vi "createPlatformDataV1.vi"() -> (3 "digital waveform":bool[](array[boolean]))   [LabVIEW 2017]
panel:
  in  "Select?":bool
  in  "Platform 61":bool
  in  "Platform 60":bool
  in  "Platform 59":bool
  in  "Platform 58":bool
  in  "Platform 57":bool
  in  "Platform 56":bool
  in  "Platform 55":bool
  in  "Platform 54":bool
  in  "Platform 53":bool
  in  "Platform 52":bool
  in  "Platform 51":bool
  in  "Platform 50":bool
  in  "Platform 49":bool
  in  "Platform 48":bool
  in  "Platform 47":bool
  in  "Platform 46":bool
  in  "Platform 45":bool
  in  "Platform 44":bool
  in  "Platform 43":bool
  in  "Platform 42":bool
  in  "Platform 41":bool
  in  "Platform 40":bool
  in  "Platform 39":bool
  in  "Platform 38":bool
  in  "Platform 37":bool
  in  "Platform 36":bool
  in  "Platform 35":bool
  in  "Platform 34":bool
  in  "Platform 33":bool
  in  "Platform 32":bool
  in  "Platform 31":bool
  in  "Platform 30":bool
  in  "Platform 29":bool
  in  "Platform 28":bool
  in  "Platform 27":bool
  in  "Platform 26":bool
  in  "Platform 25":bool
  in  "Platform 24":bool
  in  "Platform 23":bool
  in  "Platform 22":bool
  in  "Platform 21":bool
  in  "Platform 20":bool
  in  "Platform 19":bool
  in  "Platform 18":bool
  in  "Platform 17":bool
  in  "Platform 16":bool
  in  "Platform 15":bool
  in  "Platform 14":bool
  in  "Platform 13":bool
  in  "Platform 12":bool
  in  "Platform 11":bool
  in  "Platform 10":bool
  in  "Platform 9":bool
  in  "Platform 8":bool
  in  "Platform 7":bool
  in  "Platform 6":bool
  in  "Platform 5":bool
  in  "Platform 4":bool
  in  "Platform 3":bool
  in  "Platform 2":bool
  in  "Platform 1":bool
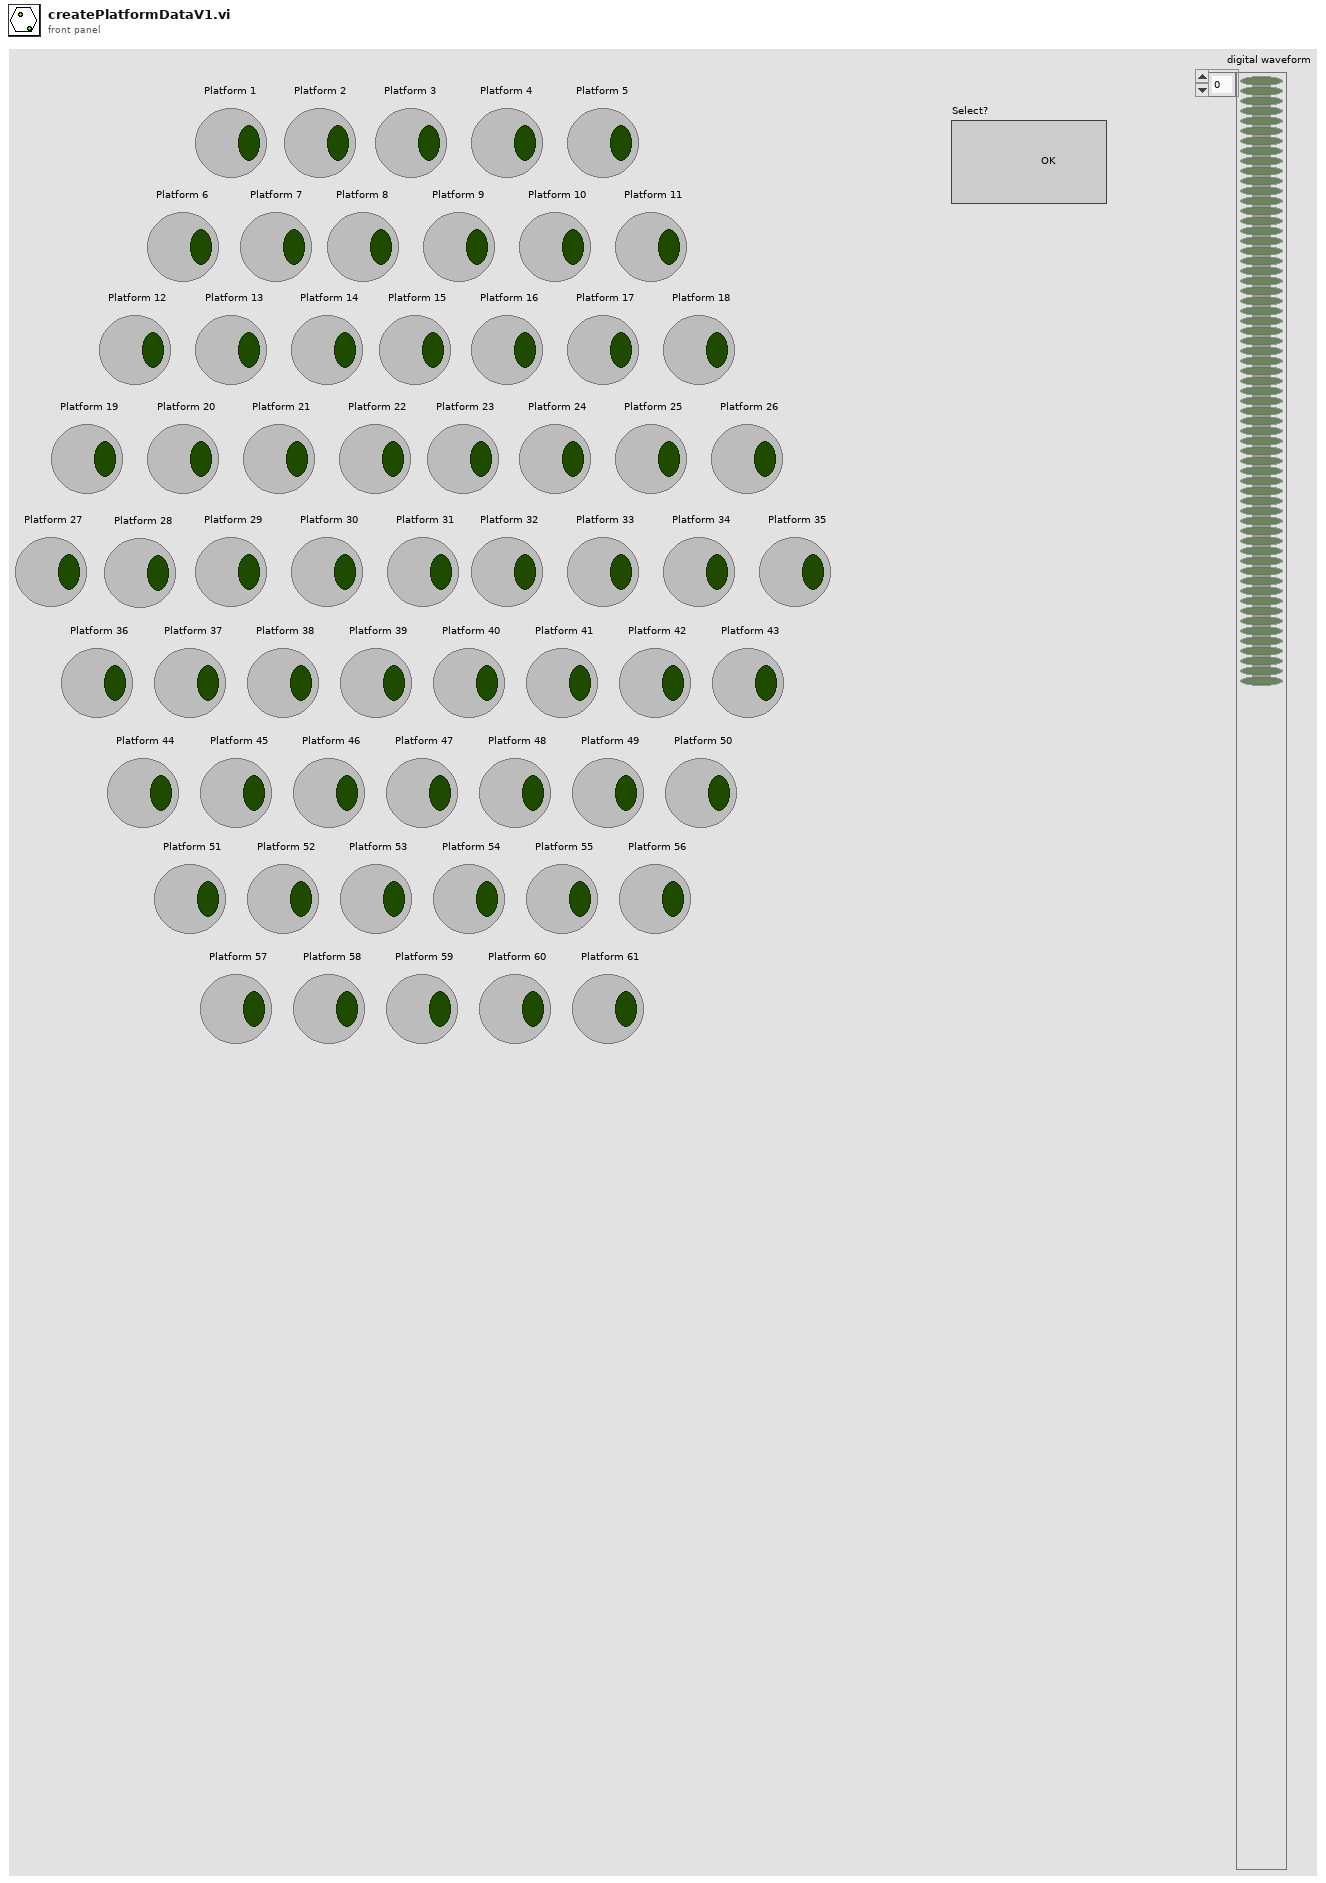
[diagram p1: front panel]
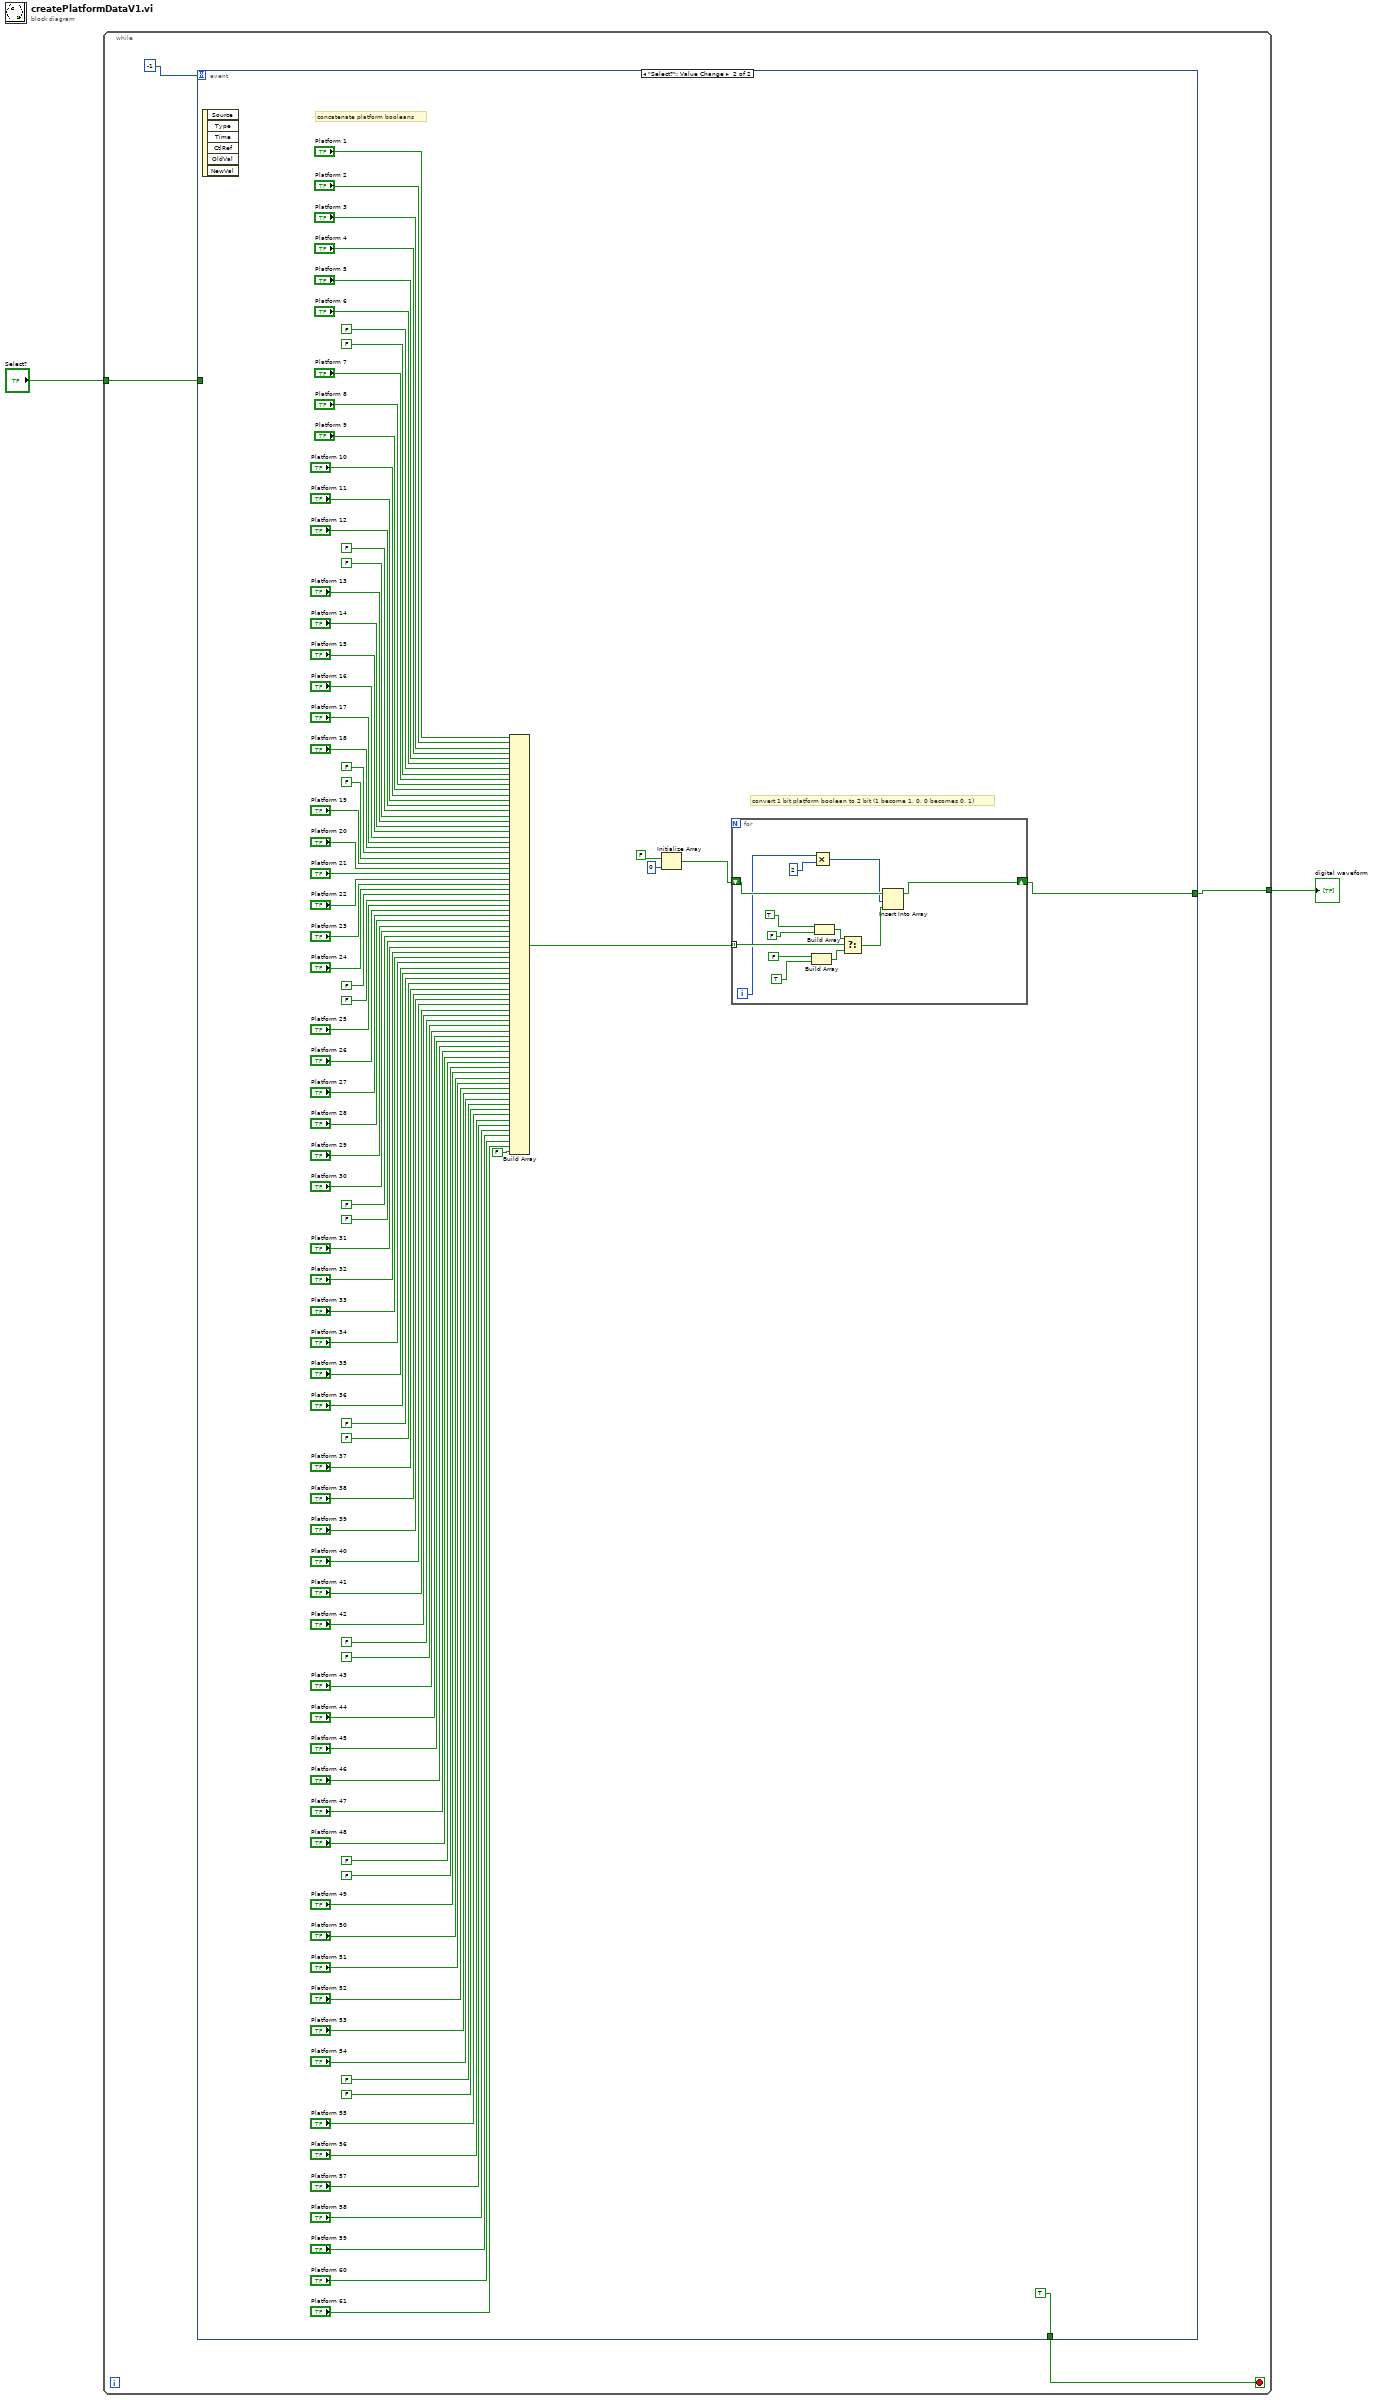
[diagram p0: block diagram]
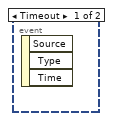
[diagram p2: hidden frame]
diagram:
  n1 = while {
    tunnel: "Select?" -> [w5]
    tunnel: [w3] -> w1
    stop <- w4 stop-if-true
    n2 = event shown="[1] \"Select?\": Value Change" {
      selector: _ -> [_ _]
      dyn-events: _ -> [_ _]
      timeout: -1 -> [_ _]
      tunnel: w5 -> [_ _]
      tunnel: [_ TRUE] -> w4
      tunnel: [_ w7] -> w3
      event Timeout {
        n3 = event-data() -> ()  [unwired: 1 in, 3 out]
      }
      event "Select?": Value Change {
        # "convert 1 bit platform boolean to 2 bit (1 become 1, 0, 0 becomes 0, 1)"
        # "concatenate platform booleans"
        n4 = event-data() -> ()  [unwired: 1 in, 6 out]
        n5 = Build Array("Platform 1", "Platform 2", "Platform 3", "Platform 4", "Platform 5", "Platform 6", FALSE, FALSE, "Platform 7", "Platform 8", "Platform 9", "Platform 10", "Platform 11", "Platform 12", FALSE, FALSE, "Platform 13", "Platform 14", "Platform 15", "Platform 16", "Platform 17", "Platform 18", FALSE, FALSE, "Platform 19", "Platform 20", "Platform 21", "Platform 22", "Platform 23", "Platform 24", FALSE, FALSE, "Platform 25", "Platform 26", "Platform 27", "Platform 28", "Platform 29", "Platform 30", FALSE, FALSE, "Platform 31", "Platform 32", "Platform 33", "Platform 34", "Platform 35", "Platform 36", FALSE, FALSE, "Platform 37", "Platform 38", "Platform 39", "Platform 40", "Platform 41", "Platform 42", FALSE, FALSE, "Platform 43", "Platform 44", "Platform 45", "Platform 46", "Platform 47", "Platform 48", FALSE, FALSE, "Platform 49", "Platform 50", "Platform 51", "Platform 52", "Platform 53", "Platform 54", FALSE, FALSE, "Platform 55", "Platform 56", "Platform 57", "Platform 58", "Platform 59", "Platform 60", "Platform 61", FALSE) -> (w12:bool[])
        n6 = Initialize Array(FALSE, 0 ("dimension size")) -> (w9:bool[])
        n7 = for {
          tunnel: w12 -> [w105] mode=indexing
          shift-right: [w93] -> w7
          shift-left: w9 -> [w98]
          i -> [w94]
          n8 = Build Array(FALSE, TRUE) -> (w102:bool[])
          n9 = Multiply(x=w94, y=2) -> (x*y=w96:i32)
          n10 = Build Array(TRUE, FALSE) -> (w99:bool[])
          n11 = Select(t=w99, s=w105, f=w102) -> (s? t:f=w95:bool[])
          n12 = Insert Into Array(array=w98, index=w96, new element=w95) -> (w93:bool[])
        }
      }
    }
  }
  "digital waveform" <- w1
